vi "Junk test ping commandline.vi"() -> ()   [LabVIEW 2013]
panel:
  out "error out":errorcluster
  out "Ping output":string
  in  "Ping options":string
  in  "IP Address":string="www.google.com"
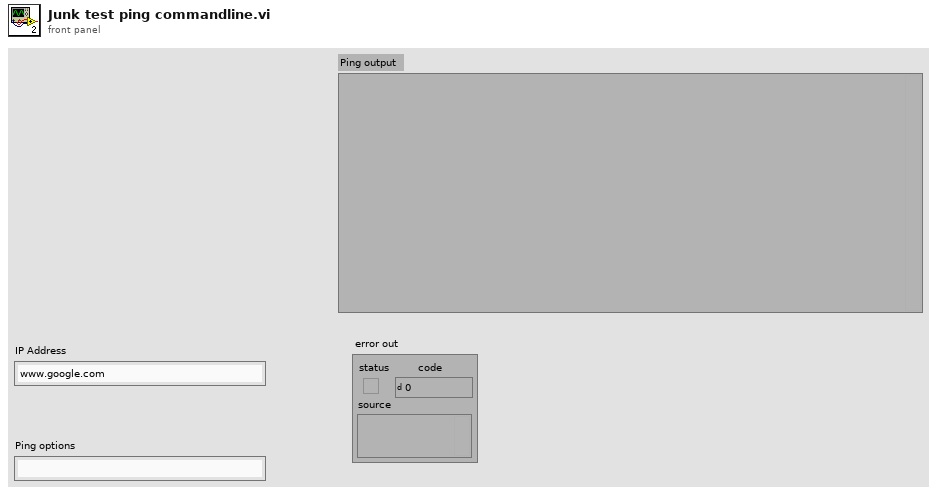
[diagram p1: front panel]
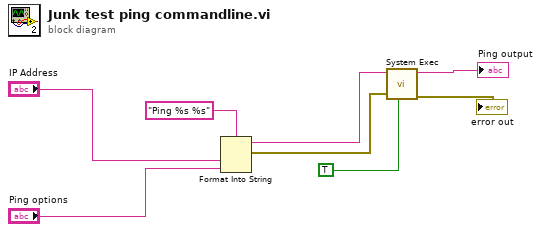
[diagram p0: block diagram]
diagram:
  n1 = Format Into String(format string="Ping %s %s", "IP Address", "Ping options") -> (resulting string=w5:string, error out=w3:errorcluster)  [unwired: 2 in]
  n2 = call <vilib>:"System Exec.vi"("run minimized? (F)"=TRUE, "error in (no error)"=w3, "command line"=w5) -> ("error out"=→"error out":errorcluster, "standard output"=→"Ping output":string)  [unwired: 5 in, 2 out]
